vi "Get Temperature.vi"(6 "Channel":i32, 8 "error in (no error)":errorcluster, 11 "Instrument.TC.MNK in":refnum<class "Inst.TC.CF.lvclass">) -> (0 "error out":errorcluster, 1 "Status":string, 2 "Temperature (K)":dbl, 3 "Instrument.TC.MNK out":refnum<class "Inst.TC.CF.lvclass">, 4 "Finished?":bool)   [LabVIEW 2019, in "Inst.TC.CF.lvclass"]
uses:
  Inst.TC.CF.lvclass
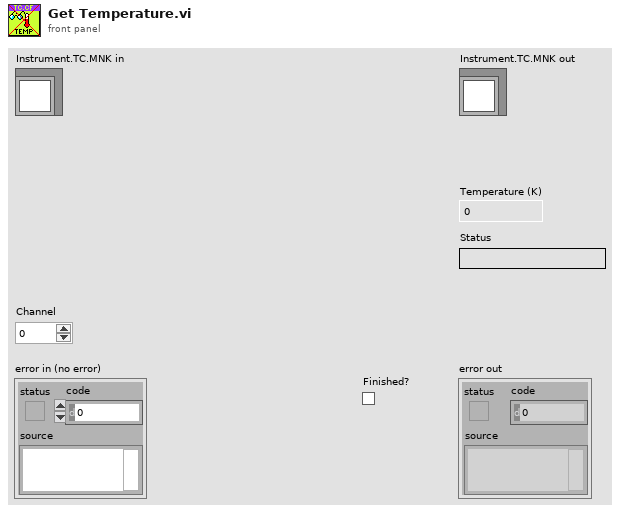
[diagram p1: front panel]
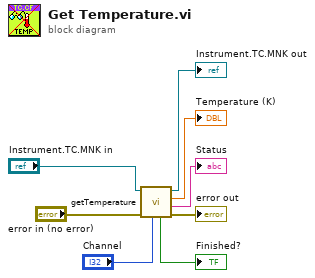
[diagram p0: block diagram]
diagram:
  n1 = call-dynamic "getTemperature.vi"("Channel"="Channel", "error in (no error)"="error in (no error)", "Instrument.TC.MNK in"="Instrument.TC.MNK in") -> ("error out"=→"error out":errorcluster, "Status"=→"Status":string, "Temperature (K)"=→"Temperature (K)":dbl, "Instrument.TC.MNK out"=→"Instrument.TC.MNK out":refnum<class "Inst.TC.CF.lvclass">, "Finished?"=→"Finished?":bool)  [unwired: 4 in]
